vi "uTTA_ucf_ReadFile_Clustered.vi"(8 "error in (no error)":errorcluster, 11 "selected path":path) -> (0 "error out":errorcluster, 2 "uTTA_Cal":T2 {"I_Sense Offset" format="%#3.3pA"; "I_Sense Gain" format="%#3.3pA/Digit"; "CH_I Offset" format="%#3.3pA"; "CH_I Gain" format="%#3.3pA/Digit"; "CH0 PA3 Offset" format="%#3.3pV"; "CH0 PA3 Gain" format="%#3.3pV/Digit"; "CH0 PA2 Offset" format="%#3.3pV"; "CH0 PA2 Gain" format="%#3.3pV/Digit"; "CH0 PA1 Offset" format="%#3.3pV"; "CH0 PA1 Gain" format="%#3.3pV/Digit"; "CH0 PA0 Offset" format="%#3.3pV"; "CH0 PA0 Gain" format="%#3.3pV/Digit"; "CH3 PA0 Offset" format="%#3.3pV"; "CH3 PA0 Gain" format="%#3.3pV/Digit"; "CH2 PA0 Offset" format="%#3.3pV"; "CH2 PA0 Gain" format="%#3.3pV/Digit"; "CH1 PA0 Offset" format="%#3.3pV"; "CH1 PA0 Gain" format="%#3.3pV/Digit"; "Voffs1 Offset" format="%#3.3pV"; "Voffs1 Gain" format="%#3.3pV/Digit"; "Voffs0 Offset" format="%#3.3pV"; "CH3 Diff Gain" format="%#3.3pV/V"; "CH2 Diff Gain" format="%#3.3pV/V"; "CH1 Diff Gain" format="%#3.3pV/V"; "Voffs0 Gain" format="%#3.3pV/Digit"; "CH0 Diff Gain" format="%#3.3pV/V"}, 3 "file path":path, 4 "TC_Channels":T1(array[cluster]), 6 "TSP_Channels":T1(array[cluster]))   [LabVIEW 2021]
uses:
  CTL_uTTA_BlockDiagCal.ctl
  <vilib>/Utility/config.llb/NI_LVConfig.lvlib
panel:
  # "G0"
  # "G1"
  # "G2"
  # "G3"
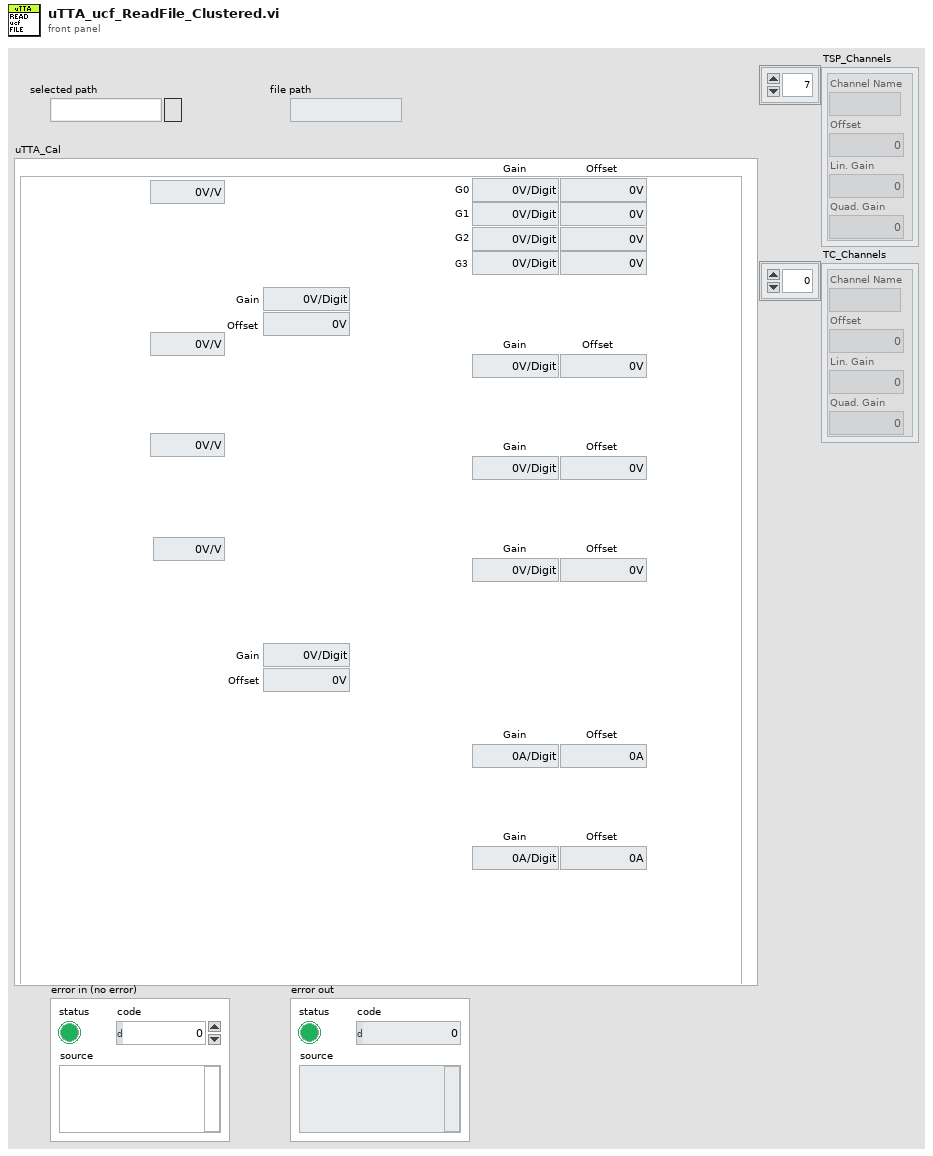
[diagram p1: front panel]
types:
  T1 = cluster{"Channel Name":string, "Offset":dbl, "Lin. Gain":dbl, "Quad. Gain":dbl}[]
  T2 = typedef "CTL_uTTA_BlockDiagCal.ctl" = cluster{"CH0 Diff Gain":dbl, "Voffs0 Gain":dbl, "CH1 Diff Gain":dbl, "CH2 Diff Gain":dbl, "CH3 Diff Gain":dbl, "Voffs0 Offset":dbl, "Voffs1 Gain":dbl, "Voffs1 Offset":dbl, "CH1 PA0 Gain":dbl, "CH1 PA0 Offset":dbl, "CH2 PA0 Gain":dbl, "CH2 PA0 Offset":dbl, "CH3 PA0 Gain":dbl, "CH3 PA0 Offset":dbl, "CH0 PA0 Gain":dbl, "CH0 PA0 Offset":dbl, "CH0 PA1 Gain":dbl, "CH0 PA1 Offset":dbl, "CH0 PA2 Gain":dbl, "CH0 PA2 Offset":dbl, "CH0 PA3 Gain":dbl, "CH0 PA3 Offset":dbl, "CH_I Gain":dbl, "CH_I Offset":dbl, "I_Sense Gain":dbl, "I_Sense Offset":dbl}
  T3 = typedef "NI_LVConfig.lvlib/Config Data RefNum.ctl" = refnum<k1>
  T4 = cluster{"Channel Name":string, "Offset":dbl, "Lin. Gain":dbl, "Quad. Gain":dbl}
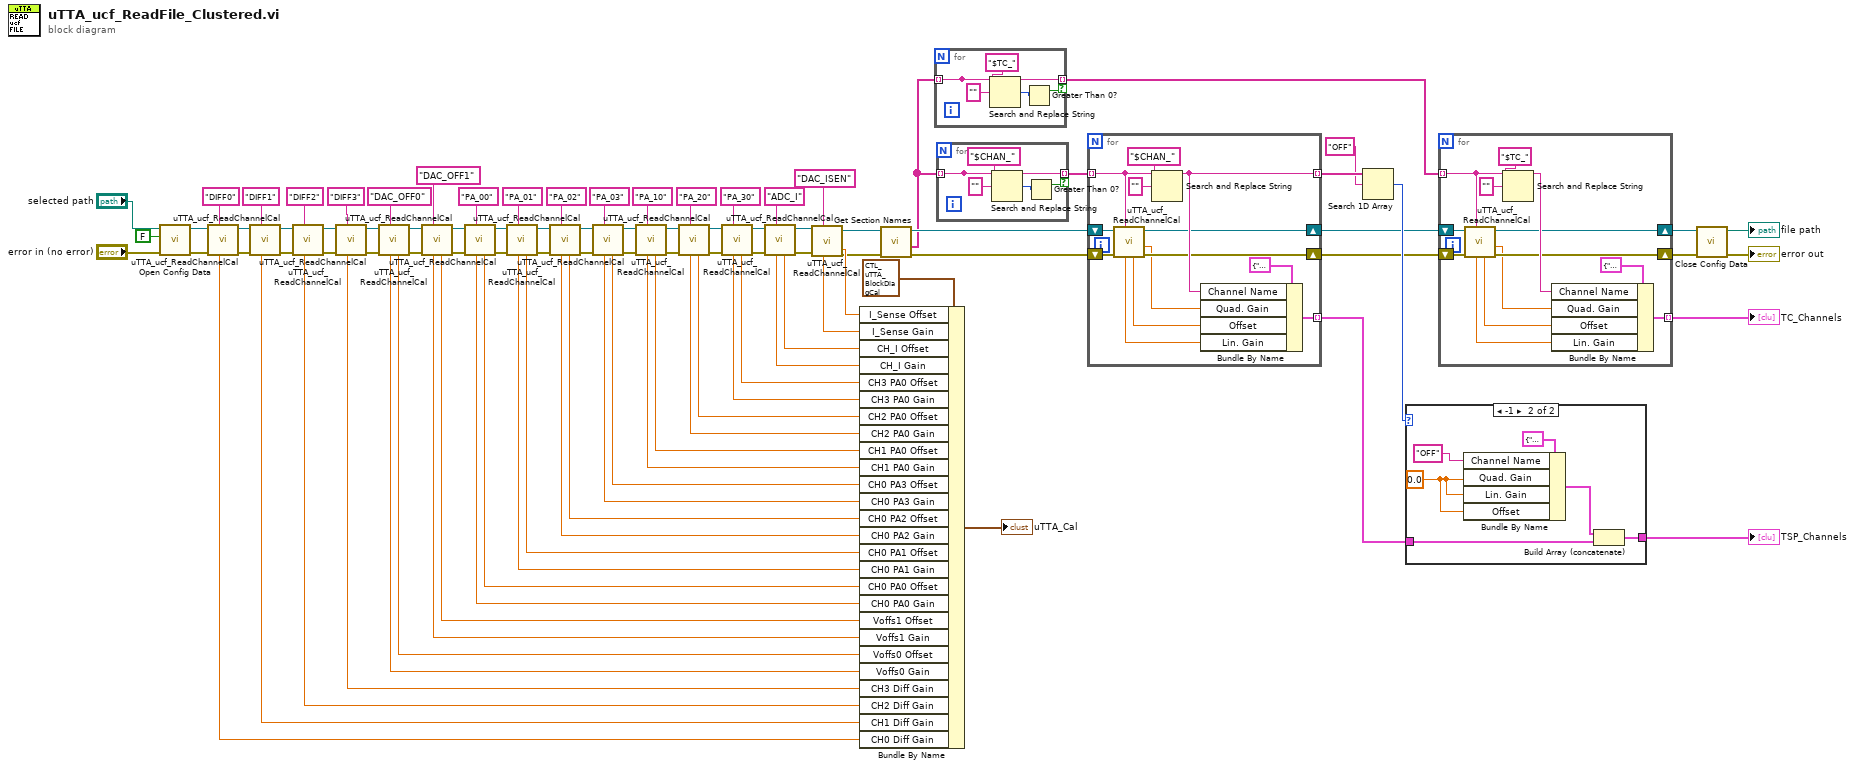
[diagram p0: block diagram]
diagram:
  n1 = call <vilib>:"Open Config Data.vi"("error in (no error)"="error in (no error)", "create file if necessary (T)"=FALSE, "configuration file path"="selected path") -> ("error out"=w24:errorcluster, "refnum"=w25:T3)  [unwired: 6 in, 1 out]
  n2 = call "uTTA_ucf_ReadChannelCal.vi"("Section"="DIFF0" ("section"), "error in"=w24, "Refnum in"=w25) -> ("error out"=w28:errorcluster, "Refnum out"=w29:T3, "LinGain"=w69:dbl)  [unwired: 4 in, 2 out]
  n3 = call "uTTA_ucf_ReadChannelCal.vi"("Section"="DIFF1" ("section"), "error in"=w28, "Refnum in"=w29) -> ("error out"=w30:errorcluster, "Refnum out"=w31:T3, "LinGain"=w70:dbl)  [unwired: 4 in, 2 out]
  n4 = call "uTTA_ucf_ReadChannelCal.vi"("Section"="DIFF2" ("section"), "error in"=w30, "Refnum in"=w31) -> ("error out"=w32:errorcluster, "Refnum out"=w33:T3, "LinGain"=w71:dbl)  [unwired: 4 in, 2 out]
  n5 = call "uTTA_ucf_ReadChannelCal.vi"("Section"="DIFF3" ("section"), "error in"=w32, "Refnum in"=w33) -> ("error out"=w34:errorcluster, "Refnum out"=w35:T3, "LinGain"=w72:dbl)  [unwired: 4 in, 2 out]
  n6 = call "uTTA_ucf_ReadChannelCal.vi"("Section"="DAC_OFF0", "error in"=w34, "Refnum in"=w35) -> ("error out"=w36:errorcluster, "Refnum out"=w37:T3, "Offset"=w74:dbl, "LinGain"=w73:dbl)  [unwired: 4 in, 1 out]
  n7 = call "uTTA_ucf_ReadChannelCal.vi"("Section"="DAC_OFF1", "error in"=w36, "Refnum in"=w37) -> ("error out"=w38:errorcluster, "Refnum out"=w39:T3, "Offset"=w76:dbl, "LinGain"=w75:dbl)  [unwired: 4 in, 1 out]
  n8 = call "uTTA_ucf_ReadChannelCal.vi"("Section"="PA_00", "error in"=w38, "Refnum in"=w39) -> ("error out"=w40:errorcluster, "Refnum out"=w41:T3, "Offset"=w78:dbl, "LinGain"=w77:dbl)  [unwired: 4 in, 1 out]
  n9 = call "uTTA_ucf_ReadChannelCal.vi"("Section"="PA_01", "error in"=w40, "Refnum in"=w41) -> ("error out"=w42:errorcluster, "Refnum out"=w43:T3, "Offset"=w80:dbl, "LinGain"=w79:dbl)  [unwired: 4 in, 1 out]
  n10 = call "uTTA_ucf_ReadChannelCal.vi"("Section"="PA_02", "error in"=w42, "Refnum in"=w43) -> ("error out"=w48:errorcluster, "Refnum out"=w49:T3, "Offset"=w82:dbl, "LinGain"=w81:dbl)  [unwired: 4 in, 1 out]
  n11 = call "uTTA_ucf_ReadChannelCal.vi"("Section"="PA_03", "error in"=w48, "Refnum in"=w49) -> ("error out"=w47:errorcluster, "Refnum out"=w50:T3, "Offset"=w84:dbl, "LinGain"=w83:dbl)  [unwired: 4 in, 1 out]
  n12 = call "uTTA_ucf_ReadChannelCal.vi"("Section"="PA_10", "error in"=w47, "Refnum in"=w50) -> ("error out"=w46:errorcluster, "Refnum out"=w51:T3, "Offset"=w86:dbl, "LinGain"=w85:dbl)  [unwired: 4 in, 1 out]
  n13 = call "uTTA_ucf_ReadChannelCal.vi"("Section"="PA_20", "error in"=w46, "Refnum in"=w51) -> ("error out"=w45:errorcluster, "Refnum out"=w52:T3, "Offset"=w88:dbl, "LinGain"=w87:dbl)  [unwired: 4 in, 1 out]
  n14 = call "uTTA_ucf_ReadChannelCal.vi"("Section"="PA_30", "error in"=w45, "Refnum in"=w52) -> ("error out"=w44:errorcluster, "Refnum out"=w53:T3, "Offset"=w90:dbl, "LinGain"=w89:dbl)  [unwired: 4 in, 1 out]
  n15 = call "uTTA_ucf_ReadChannelCal.vi"("Section"="ADC_I", "error in"=w44, "Refnum in"=w53) -> ("error out"=w22:errorcluster, "Refnum out"=w21:T3, "Offset"=w92:dbl, "LinGain"=w91:dbl)  [unwired: 4 in, 1 out]
  n16 = call "uTTA_ucf_ReadChannelCal.vi"("Section"="DAC_ISEN", "error in"=w22, "Refnum in"=w21) -> ("error out"=w2:errorcluster, "Refnum out"=w1:T3, "Offset"=w19:dbl, "LinGain"=w20:dbl)  [unwired: 4 in, 1 out]
  n17 = Bundle By Name(cluster=T2 {"CH0 Diff Gain"=123.123, "Voffs0 Gain"=123.123, "CH1 Diff Gain"=123.123, "CH2 Diff Gain"=123.123, "CH3 Diff Gain"=123.123, "Voffs0 Offset"=123.123, "Voffs1 Gain"=123.123, "Voffs1 Offset"=123.123, "CH1 PA0 Gain"=123.123, "CH1 PA0 Offset"=123.123, "CH2 PA0 Gain"=123.123, "CH2 PA0 Offset"=123.123, "CH3 PA0 Gain"=123.123, "CH3 PA0 Offset"=123.123, "CH0 PA0 Gain"=123.123, "CH0 PA0 Offset"=123.123, "CH0 PA1 Gain"=123.123, "CH0 PA1 Offset"=123.123, "CH0 PA2 Gain"=123.123, "CH0 PA2 Offset"=123.123, "CH0 PA3 Gain"=123.123, "CH0 PA3 Offset"=123.123, "CH_I Gain"=123.123, "CH_I Offset"=123.123, "I_Sense Gain"=0.0, "I_Sense Offset"=0.0} ("Inputs"), "I_Sense Offset"=w19, "I_Sense Gain"=w20, "CH_I Offset"=w92, "CH_I Gain"=w91, "CH3 PA0 Offset"=w90, "CH3 PA0 Gain"=w89, "CH2 PA0 Offset"=w88, "CH2 PA0 Gain"=w87, "CH1 PA0 Offset"=w86, "CH1 PA0 Gain"=w85, "CH0 PA3 Offset"=w84, "CH0 PA3 Gain"=w83, "CH0 PA2 Offset"=w82, "CH0 PA2 Gain"=w81, "CH0 PA1 Offset"=w80, "CH0 PA1 Gain"=w79, "CH0 PA0 Offset"=w78, "CH0 PA0 Gain"=w77, "Voffs1 Offset"=w76, "Voffs1 Gain"=w75, "Voffs0 Offset"=w74, "Voffs0 Gain"=w73, "CH3 Diff Gain"=w72, "CH2 Diff Gain"=w71, "CH1 Diff Gain"=w70, "CH0 Diff Gain"=w69) -> (→"uTTA_Cal":T2)
  n18 = call <vilib>:"Get Section Names.vi"("error in (no error)"=w2, "refnum"=w1) -> ("error out"=w15:errorcluster, "section names"=w9:string[], "refnum out"=w16:T3)  [unwired: 7 in]
  n19 = for {
    tunnel: w9 -> [w96] mode=indexing
    tunnel: [w96] -> w8 mode=indexing if=w97
    n20 = Search and Replace String(input string=w96, search string="$TC_" ("string"), replace string="" ("replace string (\"\")")) -> (number of replacements=w98:i32)  [unwired: 5 in, 3 out]
    n21 = Greater Than 0?(x=w98) -> (x > 0?=w97:bool)
  }
  n22 = for {
    tunnel: w9 -> [w101] mode=indexing
    tunnel: [w101] -> w17 mode=indexing if=w102
    n23 = Search and Replace String(input string=w101, search string="$CHAN_" ("string"), replace string="" ("replace string (\"\")")) -> (number of replacements=w103:i32)  [unwired: 5 in, 3 out]
    n24 = Greater Than 0?(x=w103) -> (x > 0?=w102:bool)
  }
  n25 = for {
    shift-right: [w111] -> w6
    shift-left: w16 -> [w113]
    shift-right: [w110] -> w7
    shift-left: w15 -> [w112]
    tunnel: w17 -> [w109] mode=indexing
    tunnel: [w117] -> w14 mode=indexing
    tunnel: [w114] -> w13 mode=indexing
    n26 = call "uTTA_ucf_ReadChannelCal.vi"("Section"=w109, "error in"=w112, "Refnum in"=w113) -> ("error out"=w110:errorcluster, "QuadGain"=w108:dbl, "Refnum out"=w111:T3, "Offset"=w107:dbl, "LinGain"=w106:dbl)  [unwired: 4 in]
    n27 = Search and Replace String(input string=w109, search string="$CHAN_" ("string"), replace string="" ("replace string (\"\")")) -> (result string=w114:string)  [unwired: 5 in, 3 out]
    n28 = Bundle By Name(cluster=T4 {"Channel Name"="", "Offset"=0.0, "Lin. Gain"=0.0, "Quad. Gain"=0.0} ("input cluster"), "Channel Name"=w114, "Quad. Gain"=w108, "Offset"=w107, "Lin. Gain"=w106) -> (w117:T4)
  }
  n29 = Search 1D Array(1D array=w13, element="OFF") -> (index of element=w11:i32)  [unwired: 1 in]
  n30 = case shown="-1" w11 {
    tunnel: w14 -> [w119 w125]
    tunnel: [w119 w124] -> w10
    frame 0, Default {
    }
    frame -1 {
      w121 = 0.0 ("Quad. Gain")
      n31 = Bundle By Name(cluster=T4 {"Channel Name"="", "Offset"=0.0, "Lin. Gain"=0.0, "Quad. Gain"=0.0} ("input cluster"), "Channel Name"="OFF", "Quad. Gain"=w121, "Lin. Gain"=w121, "Offset"=w121) -> (w120:T4)
      n32 = Build Array (concatenate)(w120, w125) -> (w124:T1)
    }
  }
  "TSP_Channels" <- w10
  n33 = for {
    shift-right: [w131] -> w3
    shift-left: w6 -> [w133]
    shift-right: [w130] -> w4
    shift-left: w7 -> [w132]
    tunnel: w8 -> [w129] mode=indexing
    tunnel: [w137] -> w5 mode=indexing
    n34 = call "uTTA_ucf_ReadChannelCal.vi"("Section"=w129, "error in"=w132, "Refnum in"=w133) -> ("error out"=w130:errorcluster, "QuadGain"=w128:dbl, "Refnum out"=w131:T3, "Offset"=w127:dbl, "LinGain"=w126:dbl)  [unwired: 4 in]
    n35 = Search and Replace String(input string=w129, search string="$TC_" ("string"), replace string="" ("replace string (\"\")")) -> (result string=w134:string)  [unwired: 5 in, 3 out]
    n36 = Bundle By Name(cluster=T4 {"Channel Name"="", "Offset"=0.0, "Lin. Gain"=0.0, "Quad. Gain"=0.0} ("input cluster"), "Channel Name"=w134, "Quad. Gain"=w128, "Offset"=w127, "Lin. Gain"=w126) -> (w137:T4)
  }
  "TC_Channels" <- w5
  n37 = call <vilib>:"Close Config Data.vi"("error in (no error)"=w4, "refnum"=w3) -> ("error out"=→"error out":errorcluster, "file path"=→"file path":path)  [unwired: 8 in]
